vi "FRCts20_Backend_Team_PUT.vi"(6 "Message Attributes":T4, 8 "error in (no error)":errorcluster, 10 "Data":string, 11 "Engine_Refnums":T1) -> (0 "error out":errorcluster)   [LabVIEW 2014, in "FRCts20_Backend_Engine.lvlib"]
doc: "Changes a team's information, called by the Team API. Expects all team information (number, name, etc.)"
uses:
  FRCts20_Backend_Engine.lvlib
  Dependencies/Keyed Array/KeyedArray.ctl
  FRCts20_Backend_EngineRefnums.ctl
  INI_Accessor/FRCts20_Backend_INI Controller.lvclass
  Dependencies/AMC/_SubVIs/TypeDefs/Message Queue.ctl
  Dependencies/AMC/_SubVIs/TypeDefs/Message.ctl
  <vilib>/addons/database/Connection.llb/Conn ObjectReference.ctl
  FRCts20_Backend_FGVOperation.ctl
  FRCts20_Backend_API/FRCts20_Backend_API_Team.ctl
  FRCts20_Backend_API/FRCts20_Backend_API_SW.ctl
  FRCts20_Backend_API/FRCts20_Backend_API_Status.ctl
  FRCts20_Backend_API/FRCts20_Backend_API.lvlib
  Dependencies/Keyed Array/Tools_KeyedArray.lvlib
  Dependencies/AMC/AMC.lvlib
  <vilib>/addons/database/NI_Database_API.lvlib
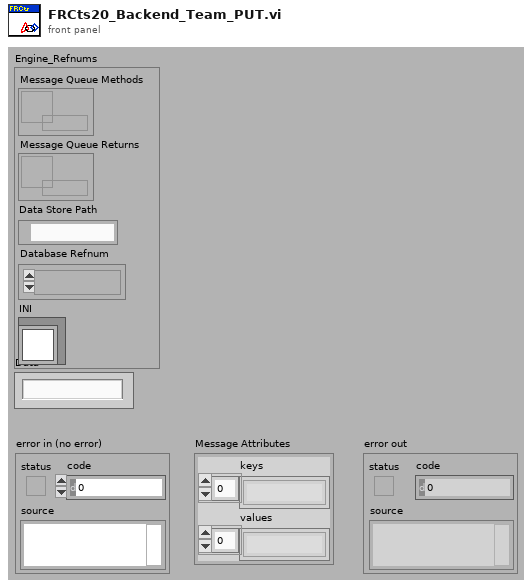
[diagram p1: front panel]
types:
  T1 = typedef "FRCts20_Backend_Engine.lvlib/FRCts20_Backend_EngineRefnums.ctl" = cluster{"Message Queue Methods":T2, "Message Queue Returns":T2, "Data Store Path":path, "Database Refnum":T3, "INI":refnum<class "FRCts20_Backend_INI Controller.lvclass">}
  T2 = typedef "AMC.lvlib/Message Queue.ctl" = refnum<queue>
  T3 = typedef "NI_Database_API.lvlib/Conn ObjectReference.ctl" = refnum<k1>
  T4 = typedef "Tools_KeyedArray.lvlib/KeyedArray.ctl" = cluster{"keys":string[], "values":string[]}
  T5 = typedef "FRCts20_Backend_API.lvlib/FRCts20_Backend_API_Team.ctl" = cluster{"Team Index":u32, "Team Number":u32, "Team Name":string, "Short Team Name":string, "Nick Name":string, "Robot Name":string, "City":string, "State":string, "Country":string, "Rookie Year":u32, "SWType":T6, "CAN":bool, "Vision":bool, "Kinect":bool, "Tags":string, "Avatar":string, "Request Array":cluster{"Request Index":u32, "Description":string, "Status":T7, "Open Date":timestamp, "Last Update":timestamp, "Close Date":timestamp}[], "Events Attending":cluster{"EventIndex":dbl, "EventName":string, "IsLive":bool}[], "APIReturn":string}
  T6 = typedef "FRCts20_Backend_API.lvlib/FRCts20_Backend_API_SW.ctl" = string
  T7 = typedef "FRCts20_Backend_API.lvlib/FRCts20_Backend_API_Status.ctl" = enum16{"Open", "In Work", "Closed"}
  T8 = typedef "FRCts20_Backend_Engine.lvlib/FRCts20_Backend_FGVOperation.ctl" = enum16{"Initialize", "EnqueueMessage", "EnqueueDataReturn", "FlushMessage", "FlushDataReturn"}
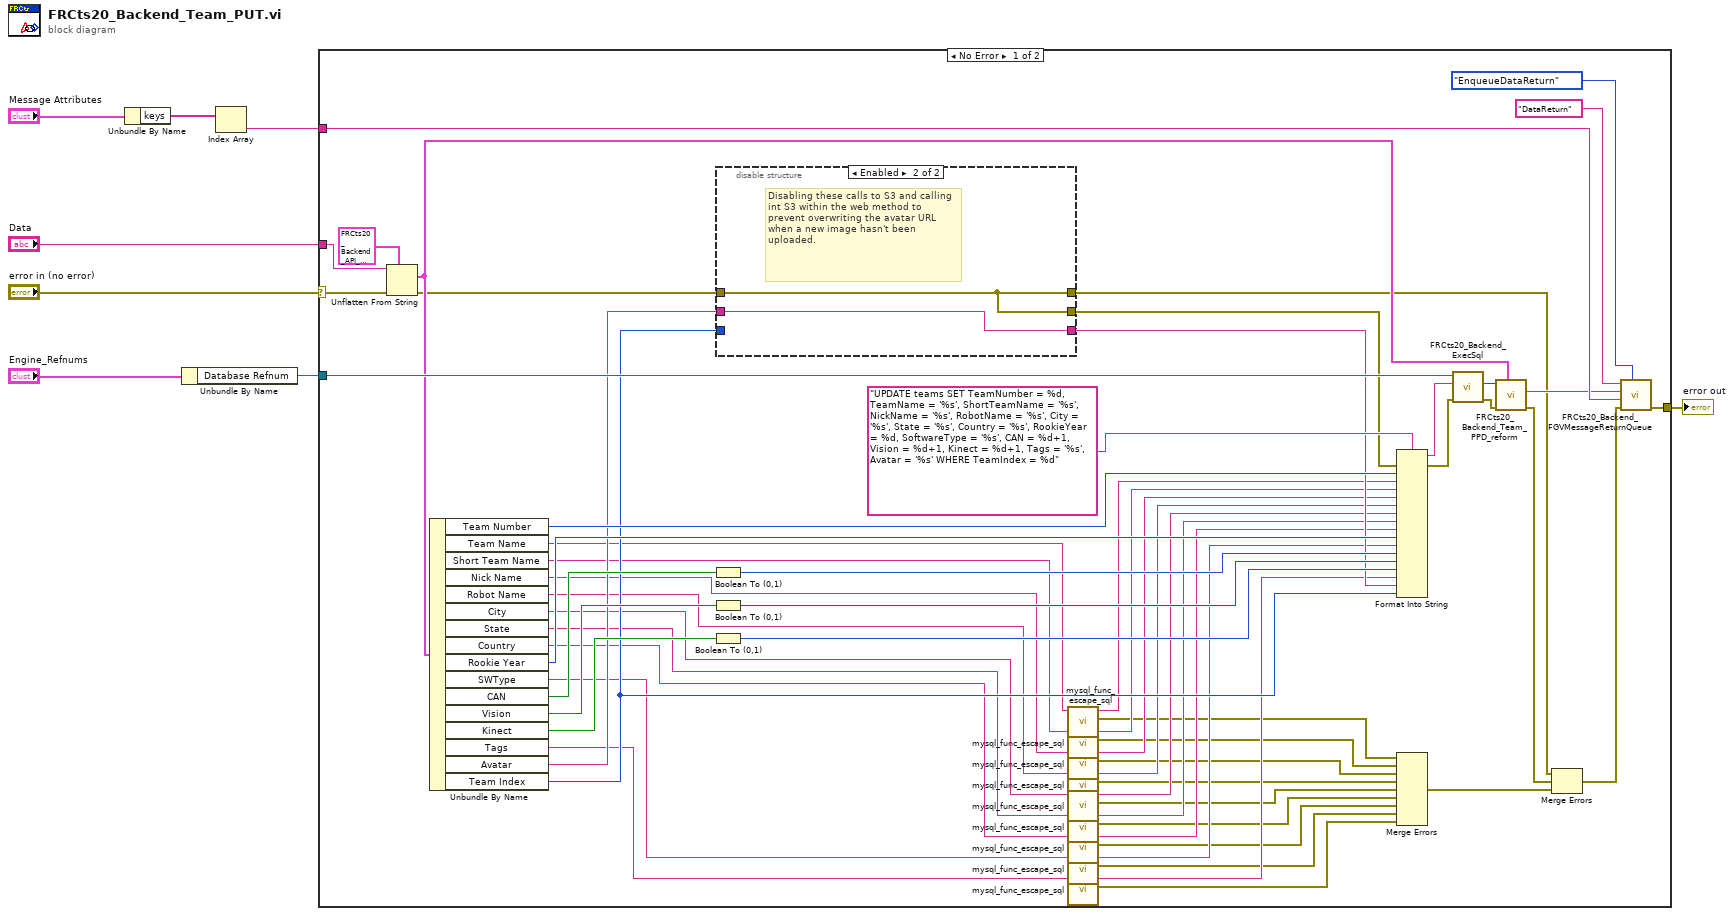
[diagram p0: block diagram]
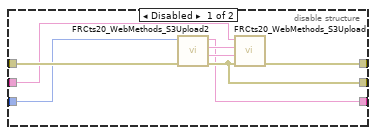
[diagram p2: hidden frame]
diagram:
  n1 = Unbundle By Name("Message Attributes") -> ("keys"=w2:string[])
  n2 = Unbundle By Name("Engine_Refnums") -> ("Database Refnum"=w5:T3)
  n3 = Index Array(array=w2) -> (element=w1:string)  [unwired: 1 in]
  n4 = case shown="No Error" "error in (no error)" {
    selector: "error in (no error)" -> [w65 w78]
    tunnel: [w37 w78] -> w7
    tunnel: w5 -> [w59 _]
    tunnel: "Data" -> [w66 _]
    tunnel: w1 -> [w67 _]
    frame No Error {
      n5 = Unflatten From String(type=T5 {"Team Index"=0, "Team Number"=0, "Team Name"="", "Short Team Name"="", "Nick Name"="", "Robot Name"="", "City"="", "State"="", "Country"="", "Rookie Year"=0, "SWType"="", "CAN"=FALSE, "Vision"=FALSE, "Kinect"=FALSE, "Tags"="", "Avatar"="", "Request Array"=[], "Events Attending"=[], "APIReturn"=""} ("Team"), binary string=w66, error in (no error)=w65) -> (value=w50:T5, error out=w44:errorcluster)  [unwired: 2 in, 1 out]
      n6 = Unbundle By Name(w50) -> ("Team Number"=w57:u32, "Team Name"=w36:string, "Short Team Name"=w34:string, "Nick Name"=w33:string, "Robot Name"=w32:string, "City"=w31:string, "State"=w30:string, "Country"=w29:string, "Rookie Year"=w56:u32, "SWType"=w28:T6, "CAN"=w55:bool, "Vision"=w52:bool, "Kinect"=w53:bool, "Tags"=w20:string, "Avatar"=w43:string, "Team Index"=w40:u32)
      n7 = Boolean To (0,1)(Boolean=w55) -> (0, 1=w54:i16)
      n8 = Boolean To (0,1)(Boolean=w52) -> (0, 1=w51:i16)
      n9 = Boolean To (0,1)(Boolean=w53) -> (0, 1=w46:i16)
      n10 = disable-structure shown="Enabled" {
        disable-tunnel: [w75 w76] -> w45
        disable-tunnel: w44 -> [w74 w76]
        disable-tunnel: w43 -> [w73 w77]
        disable-tunnel: [w72 w76] -> w42
        disable-tunnel: [w69 w77] -> w41
        disable-tunnel: w40 -> [w68 _]
        frame Disabled {
          n11 = call "FRCts20_WebMethods_S3Upload2.vi"("error in (no error)"=w74, "Team Index"=w68) -> ("error out"=w72:errorcluster, "Bucket"=w70:string, "Object Path"=w71:string, "S3 URL"=w69:string)  [unwired: 6 in]
          n12 = call "FRCts20_WebMethods_S3Upload.vi"("error in (no error)"=w72, "Bucket"=w70, "Object Path"=w71, "Temporary URL"=w73) -> ("error out"=w75:errorcluster)  [unwired: 7 in]
        }
        frame Enabled {
          # "Disabling these calls to S3 and calling int S3 within the web method to prevent overwriting the avatar URL when a new image hasn't been uploaded."
        }
      }
      n13 = call "mysql_func_escape_sql.vi"("sqlin"=w36) -> ("error out"=w18:errorcluster, "escaped"=w35:string)  [unwired: 9 in]
      n14 = call "mysql_func_escape_sql.vi"("sqlin"=w34) -> ("error out"=w17:errorcluster, "escaped"=w27:string)  [unwired: 9 in]
      n15 = call "mysql_func_escape_sql.vi"("sqlin"=w33) -> ("error out"=w16:errorcluster, "escaped"=w26:string)  [unwired: 9 in]
      n16 = call "mysql_func_escape_sql.vi"("sqlin"=w32) -> ("error out"=w15:errorcluster, "escaped"=w25:string)  [unwired: 9 in]
      n17 = call "mysql_func_escape_sql.vi"("sqlin"=w31) -> ("error out"=w14:errorcluster, "escaped"=w24:string)  [unwired: 9 in]
      n18 = call "mysql_func_escape_sql.vi"("sqlin"=w30) -> ("error out"=w13:errorcluster, "escaped"=w23:string)  [unwired: 9 in]
      n19 = call "mysql_func_escape_sql.vi"("sqlin"=w29) -> ("error out"=w12:errorcluster, "escaped"=w22:string)  [unwired: 9 in]
      n20 = call "mysql_func_escape_sql.vi"("sqlin"=w28) -> ("error out"=w11:errorcluster, "escaped"=w21:string)  [unwired: 9 in]
      n21 = call "mysql_func_escape_sql.vi"("sqlin"=w20) -> ("error out"=w10:errorcluster, "escaped"=w19:string)  [unwired: 9 in]
      n22 = Format Into String(format string="UPDATE teams SET TeamNumber = %d, TeamName = '%s', ShortTeamName = '%s', NickName = '%s', RobotName = '%s', City = '%s', State = '%s', Country = '%s', RookieYear = %d, SoftwareType = '%s', CAN = %d+1, Vision = %d+1, Kinect = %d+1, Tags = '%s', Avatar = '%s' WHERE TeamIndex = %d", error in=w42, w57, w35, w27, w26, w25, w24, w23, w22, w56, w21, w54, w51, w46, w19, w41, w40) -> (resulting string=w47:string, error out=w49:errorcluster)  [unwired: 1 in]
      n23 = Merge Errors(w18, w17, w16, w15, w14, w13, w12, w11, w10) -> (w9:errorcluster)
      n24 = call "FRCts20_Backend_ExecSql.vi"("error in (no error)"=w49, "format string"=w47, "Refnum in"=w59) -> ("error out"=w60:errorcluster, "rows affected"=w61:i32)  [unwired: 6 in, 1 out]
      n25 = call "FRCts20_Backend_Team_PPD_reform.vi"("Team"=w50, "error in (no error)"=w60, "rows affected"=w61) -> ("error out"=w39:errorcluster, "data string"=w58:string)  [unwired: 7 in]
      n26 = Merge Errors(w45, w39, w9) -> (w38:errorcluster)
      n27 = call "FRCts20_Backend_FGVMessageReturnQueue.vi"("Operation"=FRCts20_Backend_FGVOperation."EnqueueDataReturn", "error in (no error)"=w38, "Key"=w67, "Message Value"=w58, "Message Name"="DataReturn") -> ("error out"=w37:errorcluster)  [unwired: 5 in, 1 out]
    }
    frame Error {
    }
  }
  "error out" <- w7
